vi "Do_Address_tl.vi"(2 "CHANNEL PARAMETERS":string[][](table), 5 "Axis Name":string) -> (1 "Current Axis Name":string)   [LabVIEW 2010]
panel:
  in  "Case Constant\n(See Context Help) 2":bool=TRUE
  in  "Case Constant\n(See Context Help)":bool=TRUE
  out "Card No.":i32
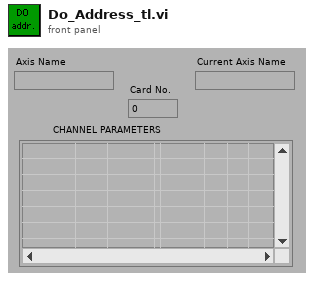
[diagram p1: front panel]
types:
  T1 = enum16{"Is Axis Current axis?", "Write Parameters", "Set Address", "Selected OK?", "Update current axis"}
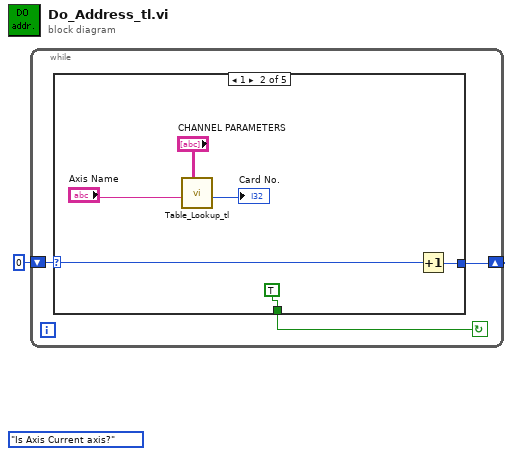
[diagram p0: block diagram]
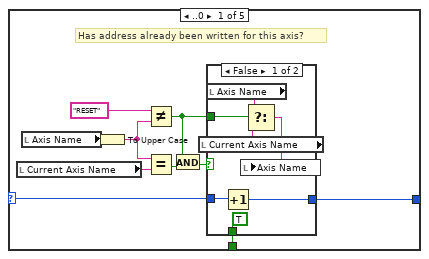
[diagram p2: hidden frame]
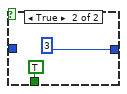
[diagram p3: hidden frame]
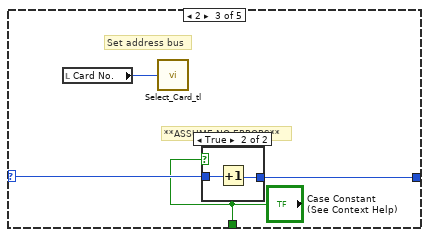
[diagram p4: hidden frame]
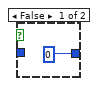
[diagram p5: hidden frame]
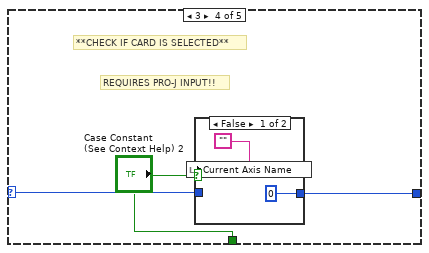
[diagram p6: hidden frame]
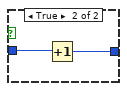
[diagram p7: hidden frame]
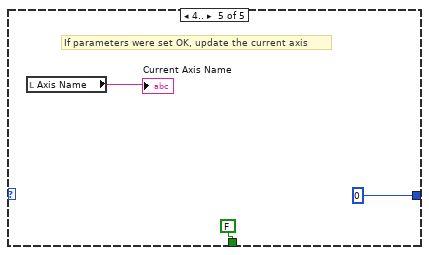
[diagram p8: hidden frame]
diagram:
  (unwired) T1."Is Axis Current axis?"
  n1 = while {
    shift-left: 0 -> [w4]
    shift-right: [w3] -> _
    stop <- w2 continue-if-true
    n2 = case shown="1" w4 {
      selector: w4 -> [w13 w29 w33 w39 _]
      tunnel: [w12 w28 w32 w38 0] -> w3
      tunnel: [w11 TRUE "Case Constant\n(See Context Help)" "Case Constant\n(See Context Help) 2" FALSE] -> w2
      frame ..0 {
        # "Has address already been written for this axis?"
        n3 = local read "Current Axis Name"() -> (w14:string)
        n4 = local read "Axis Name"() -> (w10:string)
        n5 = To Upper Case(1:w10) -> (0:w6:string)
        n6 = Not Equal?(x="RESET", y=w6) -> (x != y?=w5:bool)
        n7 = Equal?(x=w6, y=w14) -> (x = y?=w9:bool)
        n8 = And(x=w5, y=w9) -> (x .and. y?=w7:bool)
        n9 = case shown="False" w7 {
          tunnel: w13 -> [w21 _]
          tunnel: [w20 3] -> w12
          tunnel: [TRUE TRUE] -> w11
          tunnel: w5 -> [w18 _]
          frame False {
            n10 = local read "Current Axis Name"() -> (w15:string)
            n11 = local read "Axis Name"() -> (w17:string)
            n12 = Increment(x=w21) -> (x+1=w20:i32)
            n13 = Select(t=w17, s=w18, f=w15) -> (s? t:f=w16:string)
            n14 = local write "Axis Name"(w16) -> ()
          }
          frame True {
          }
        }
      }
      frame 1 {
        n15 = call "Table_Lookup_tl.vi"("Lookup Table"="CHANNEL PARAMETERS", "Search String"="Axis Name") -> ("Integer Output"=→"Card No.":i32)  [unwired: 3 in, 3 out]
        n16 = Increment(x=w29) -> (x+1=w28:i32)
      }
      frame 2 {
        # "**ASSUME NO ERRORS**"
        # "Set address bus"
        n17 = local read "Card No."() -> (w30:i32)
        n18 = call "Select_Card_tl.vi"("Card number"=w30) -> ()  [unwired: 1 in]
        n19 = case shown="True" "Case Constant\n(See Context Help)" {
          tunnel: w33 -> [_ w36]
          tunnel: [0 w35] -> w32
          frame False {
          }
          frame True {
            n20 = Increment(x=w36) -> (x+1=w35:i32)
          }
        }
      }
      frame 3 {
        # "REQUIRES PRO-J INPUT!!"
        # "**CHECK IF CARD IS SELECTED**"
        n21 = case shown="False" "Case Constant\n(See Context Help) 2" {
          tunnel: w39 -> [_ w43]
          tunnel: [0 w42] -> w38
          frame False {
            n22 = local write "Current Axis Name"("") -> ()
          }
          frame True {
            n23 = Increment(x=w43) -> (x+1=w42:i32)
          }
        }
      }
      frame 4.. {
        # "If parameters were set OK, update the current axis"
        n24 = local read "Axis Name"() -> (→"Current Axis Name":string)
      }
    }
  }
